vi "SIAMScript_to_String.vi"(8 "error in (no error)":errorcluster, 11 "Script":T2(array[cluster])=[{"Delay 10µs"=0, "command"=4027514895, "P0"=16777215, "P1"=0, "P2"=0, "P3"=0, "P4"=0, "P5-ticket"=0}, {"Delay 10µs"=0, "command"=4027514895, "P0"=100, "P1"=0, "P2"=0, "P3"=0, "P4"=0, "P5-ticket"=0}, {"Delay 10µs"=0, "command"=4027514895, "P0"=5, "P1"=120, "P2"=0, "P3"=0, "P4"=0, "P5-ticket"=0}] {"command" format="%x" items=["read_x-Motor_status_ticket"=17305600, "init_x-Motor"=17760263, "read_x-Motor_absolute_ticket"=16781312, "move_x-Motor_absolute"=16777217, "move_x-Motor_relative"=16842753, "read_y-Motor_status_ticket"=18354176, "init_y-Motor"=18808839, "read_y-Motor_absolute_ticket"=17829888, "move_y-Motor_absolute"=17825793, "move_y-Motor_relative"=17891329, "read_z-Motor_status_ticket"=19402752, "init_z-Motor"=19857415, "stop_z-Motor"=19857423, "start_z-Motor"=19857422, "read_z-Motor_absolute_ticket"=18878464, "move_z-Motor_absolute"=18874369, "move_z-Motor_relative"=18939905, "end_no_ticket"=4027514895, "end_ticket"=4027518991, "IO-read_bank0"=3489665024, "IO-write_bank0"=3489660929, "IO-read_bank1"=3506442240, "IO-write_bank1"=3506438145, "Analog-write_DA0-0"=2684354561, "Analog-write_DA0-1"=2685403137, "Analog-write_DA0-2"=2686451713, "Analog-write_DA0-3"=2687500289, "Analog-write_DA0-4"=2688548865, "Analog-write_DA0-5"=2689597441, "Analog-write_DA0-6"=2690646017, "Analog-write_DA0-7"=2691694593, "Analog-write_DA1-0"=2701131777, "Analog-write_DA1-1"=2702180353, "Analog-write_DA1-2"=2703228929, "Analog-write_DA1-3"=2704277505, "Analog-write_DA1-4"=2705326081, "Analog-write_DA1-5"=2706374657, "Analog-write_DA1-6"=2707423233, "Analog-write_DA1-7"=2708471809, "Analog-read_AD0-0"=2818576384, "Analog-read-store_AD0-0"=2818572290, "IO-delay_bank0"=3489923073, "IO-delay_bank0_fromVar"=3489923075, "read_cam_clock"=3289124864, "store_cam_clock"=3289120770, "read_cam_phase"=3289190400, "set_cam_deadtime"=3288989697, "set_cam_10uscycles"=3289055233, "set_cam_10uscycles_fromVariable"=3289055235, "calc_cam"=3289317386, "store_cam_Var"=3289251842, "math_addToVariable"=4060086278, "readVar"=4060090368, "writeVar"=4060086273, "copyVar"=4060086276, "decrement_branchRel_if_equal"=4043374945, "decrement_branchRel_if_greaterequal"=4043375201, "decrement_branchRel_if_greaterequal_withTicket"=4043379297, "decrement_branchRel_if_smaller"=4043375457, "increment_branchRel_if_smaller"=4043375473, "set_x-Galvo"=102760689, "set_y-Galvo"=103809265, "set_z-Fokus"=104857841, "set_x-Galvo_position-only"=102760513, "set_y-Galvo_position-only"=103809089, "set_z-Fokus_position-only"=104857665, "set_x-Galvo_position-only_ticket"=102764609, "set_y-Galvo_position-only_ticket"=103813185, "set_z-Fokus_position-only_ticket"=104861761, "set_x-Galvo_speed-only"=102760481, "set_y-Galvo_speed-only"=103809057, "set_z-Fokus_speed-only"=104857633, "read_x-Galvo_ticket"=102764608, "read_y-Galvo_ticket"=103813184, "read_z-Focus_ticket"=104861760, "x-Galvo_pos_fromVar"=102760515, "y-Galvo_pos_fromVar"=103809091, "z-Focus_pos_fromVar"=104857667]}) -> (0 "error out":errorcluster, 3 "String":string="00000000 0D000001 00FFFFFF 00000000 00000000 00000000 00000000 00000100\n00000000 C40A0001 00000064 00000000 00000000 00000000 00000000 00000101\n00000000 F2000001 00000057 00000078 00000000 00000000 00000000 00000102\n00000000 C40B0003 00000057 00000000 00000000 00000000 00000000 00000103\n00000001 C40F000A 00000000 00000000 00000000 00000000 00000000 00000104\n00000000 C40C1000 00000000 00000000 00000000 00000000 00000000 00000105\n00000000 C40D1000 00000000 00000000 00000000 00000000 00000000 00000106\n00000000 C40E0002 00000056 00000000 00000000 00000000 00000000 00000107\n00000000 F2000006 00000056 FFFFFFCE 00000000 00000000 00000000 00000108\n00000000 0D041003 00000056 00000000 00000000 00000000 00000000 00000109\n00000001 F1011261 00000000 00000057 00000002 00000000 00000000 0000010A\n00000000 0D000001 00000001 00000001 00000000 00000000 00000000 0000010B\n00000002 0D000001 00000001 00000000 00000000 00000000 00000000 0000010C\n00000001 F00F100F 00000000 00000000 00000000 00000000 00000000 00000FFF")   [LabVIEW 2011]
uses:
  SIAM_command.ctl
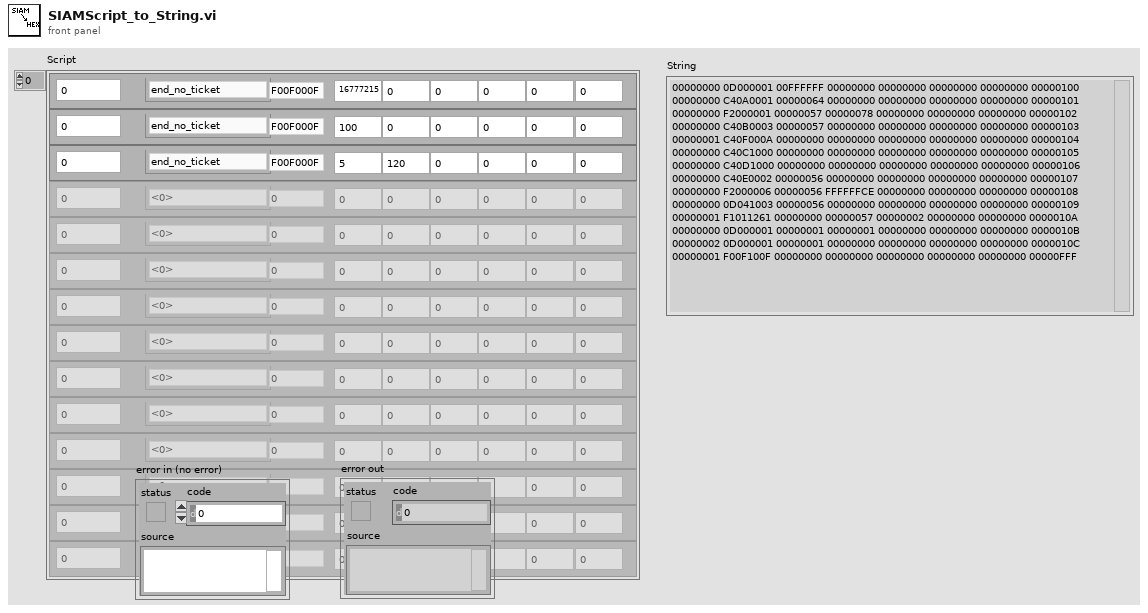
[diagram p1: front panel]
types:
  T1 = typedef "SIAM_command.ctl" = u32
  T2 = cluster{"Delay 10µs":u32, "command":T1, "P0":i32, "P1":i32, "P2":i32, "P3":i32, "P4":i32, "P5-ticket":i32}[]
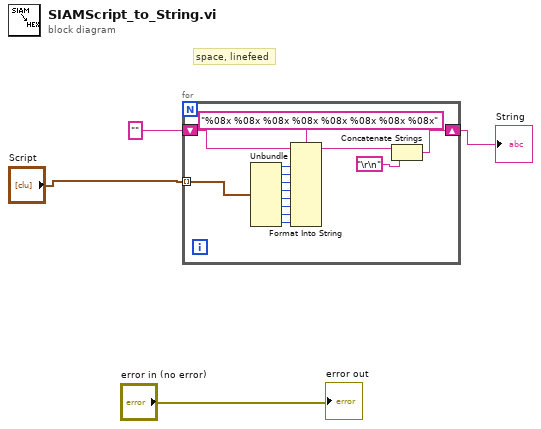
[diagram p0: block diagram]
diagram:
  # "space, linefeed"
  n1 = for {
    tunnel: "Script" -> [w18] mode=indexing
    shift-right: [w6] -> w1
    shift-left: "" -> [w7]
    n2 = Unbundle(w18) -> ("Delay 10µs"=w17:u32, "command"=w16:T1, "P0"=w15:i32, "P1"=w14:i32, "P2"=w13:i32, "P3"=w12:i32, "P4"=w11:i32, "P5-ticket"=w10:i32)
    n3 = Format Into String(format string="%08x %08x %08x %08x %08x %08x %08x %08x", initial string=w7, w17, w16, w15, w14, w13, w12, w11, w10) -> (resulting string=w8:string)  [unwired: 1 in, 1 out]
    n4 = Concatenate Strings(w8, "\r\n") -> (w6:string)
  }
  "String" <- w1
  "error out" <- "error in (no error)"
